vi "Filter IP regex.vi"(8 "error in":errorcluster, 11 "IP":string) -> (0 "Error out":errorcluster, 2 "IP Valid?":bool, 3 "Filtered IP":string)   [LabVIEW 2021, in "UDP Comms.lvlib"]
uses:
  UDP Comms.lvlib
  <vilib>/regexp/Match Regular Expression.xnode
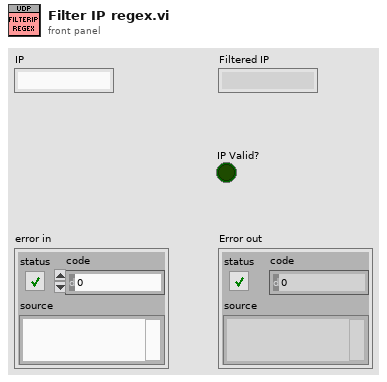
[diagram p1: front panel]
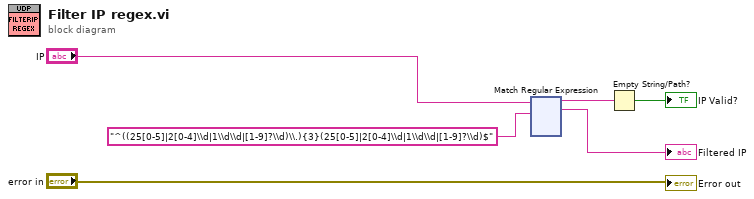
[diagram p0: block diagram]
diagram:
  n1 = xnode "Match Regular Expression"("input string"="IP", "regular expression"="^((25[0-5]|2[0-4]\\d|1\\d\\d|[1-9]?\\d)\\.){3}(25[0-5]|2[0-4]\\d|1\\d\\d|[1-9]?\\d)$") -> ("before match"=w2:string, "whole match"=→"Filtered IP":string)  [unwired: 4 in, 3 out]
  n2 = Empty String/Path?(string/path=w2) -> (empty?=→"IP Valid?":bool)
  "Error out" <- "error in"
